vi "Listbox SelMode.vi"(8 "错误输入":errorcluster, 11 "Listbox Ref":refnum<vi>) -> (0 "错误输出":errorcluster, 1 "Array?":bool, 2 "SelMode":T1, 3 "Dup Listbox Ref":refnum<vi>)   [LabVIEW 2012, in "Listbox Tool.lvlib"]
uses:
  Listbox Tool.lvlib
  Custom Type/SelMode.ctl
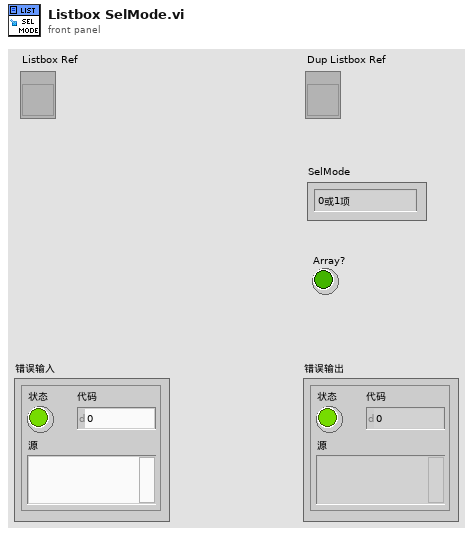
[diagram p1: front panel]
types:
  T1 = typedef "Listbox Tool.lvlib/SelMode.ctl" = enum16{"0或1项", "1项", "0或多项", "1或多项"}
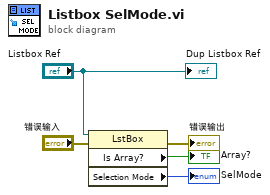
[diagram p0: block diagram]
diagram:
  n1 = property class="LstBox"(reference="Listbox Ref", error in="错误输入") -> (error out=→"错误输出":errorcluster, "Is Array?"=→"Array?":bool, "Selection Mode"=→"SelMode":i32)  [unwired: 1 out]
  "Dup Listbox Ref" <- "Listbox Ref"
